vi "Create Detrough Envelope Waveform.vi"(0 "Reference Waveform":T3 {"Runtime Scaling" format="%#_6p"; "Sample Rate" format="%#_6p"; "Burst Length (s)" format="%#_6p"; "PAPR (dB)" format="%.2f"; "Signal Bandwidth (Hz)" format="%#_6p"}, 5 "Detrough Configuration":T1={"Type"=enum."Exponential", "Minimum Voltage (V)"=1.5, "Maximum Voltage (V)"=3.5, "Exponent"=1.2000000476837158}, 11 "error in (no error)":errorcluster) -> (4 "Detrough Envelope Waveform":T3 {"Runtime Scaling" format="%#_6p"; "Sample Rate" format="%#_6p"; "Burst Length (s)" format="%#_6p"; "PAPR (dB)" format="%.2f"; "Signal Bandwidth (Hz)" format="%#_6p"}, 15 "error out":errorcluster)   [LabVIEW 2019, in "Envelope Tracking.lvlib"]
doc: "Creates an envelope waveform utilizing the detrough method."
uses:
  Envelope Tracking.lvlib
  Common/Waveform.ctl
  Typedefs/Detrough Configuration.ctl
  Typedefs/Detrough Type.ctl
  Common/Common.lvlib
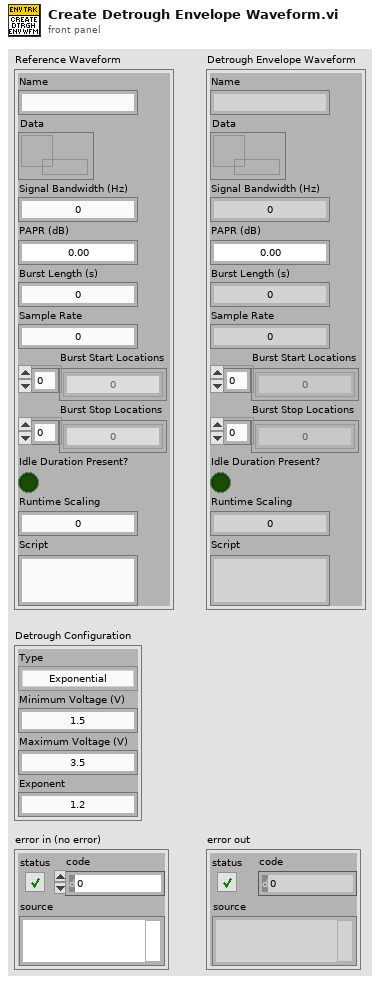
[diagram p1: front panel]
types:
  T1 = typedef "Envelope Tracking.lvlib/Detrough Configuration.ctl" = cluster{"Type":T2, "Minimum Voltage (V)":dbl, "Maximum Voltage (V)":dbl, "Exponent":dbl}
  T2 = typedef "Envelope Tracking.lvlib/Detrough Type.ctl" = enum16{"Exponential", "Cosine", "Power"}
  T3 = typedef "Common.lvlib/Waveform.ctl" = cluster{"Name":string, "Data":refnum<data-value>, "Signal Bandwidth (Hz)":dbl, "PAPR (dB)":dbl, "Burst Length (s)":dbl, "Sample Rate":dbl, "Burst Start Locations":i32[], "Burst Stop Locations":i32[], "Idle Duration Present?":bool, "Runtime Scaling":dbl, "Script":string}
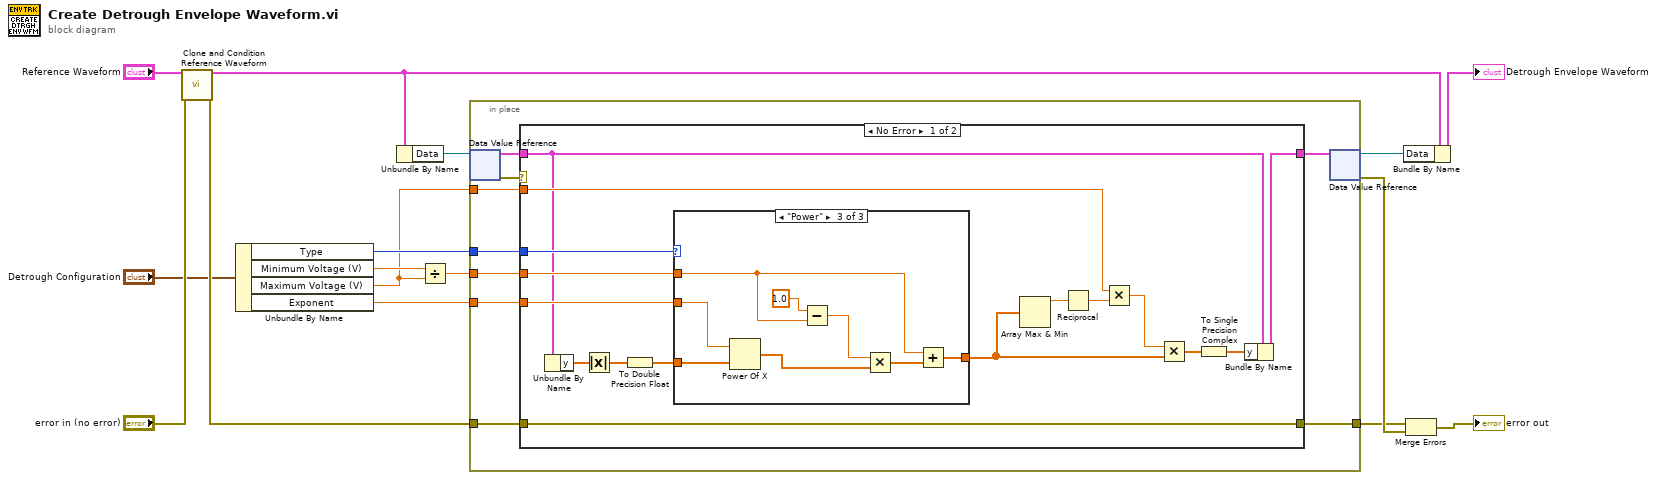
[diagram p0: block diagram]
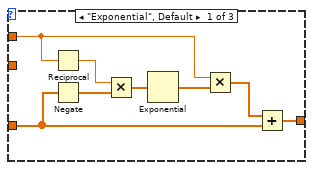
[diagram p2: hidden frame]
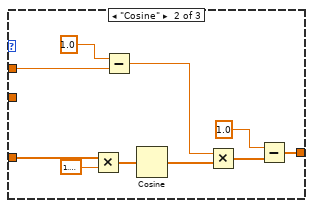
[diagram p3: hidden frame]
diagram:
  n1 = call "Clone and Condition Reference Waveform.vi"("Reference Waveform"="Reference Waveform", "error in (no error)"="error in (no error)") -> ("Conditioned Reference Waveform"=w3:T3, "error out"=w15:errorcluster)  [unwired: 12 in]
  n2 = Unbundle By Name("Detrough Configuration") -> ("Type"=w9:T2, "Minimum Voltage (V)"=w8:dbl, "Maximum Voltage (V)"=w7:dbl, "Exponent"=w6:dbl)
  n3 = Unbundle By Name(w3) -> ("Data"=w2:refnum<data-value>)
  n4 = Divide(x=w8, y=w7) -> (x/y=w10:dbl)
  n5 = in-place {
    in-place-border: w10 -> [w22]
    in-place-border: w9 -> [w21]
    in-place-border: w7 -> [w20]
    in-place-border: w6 -> [w19]
    in-place-border: w15 -> [w24]
    in-place-border: [w23] -> w13
    n6 = in-place-dvr #1(w2) -> (w18:cluster{"t0":dbl, "dt":dbl, "y":csg[]}, w25:errorcluster)
    n7 = case shown="No Error" w25 {
      tunnel: w22 -> [w38 _]
      tunnel: w21 -> [w36 _]
      tunnel: w20 -> [w35 _]
      tunnel: w19 -> [w34 _]
      tunnel: w18 -> [w27 w68]
      tunnel: [w26 w68] -> w17
      tunnel: w24 -> [w41 w69]
      tunnel: [w41 w69] -> w23
      frame No Error {
        n8 = Unbundle By Name(w27) -> ("y"=w33:csg[])
        n9 = Absolute Value(x=w33) -> (abs(x)=w31:sgl[])
        n10 = To Double Precision Float(number=w31) -> (double precision float=w30:dbl[])
        n11 = case shown="\"Power\"" w36 {
          tunnel: w30 -> [w43 w59 w67]
          tunnel: w38 -> [w45 w51 w61]
          tunnel: [w42 w54 w63] -> w32
          tunnel: w34 -> [_ _ w66]
          frame "Exponential", Default {
            n12 = Reciprocal(x=w45) -> (1/x=w47:dbl)
            n13 = Negate(x=w43) -> (-x=w49:dbl[])
            n14 = Multiply(x=w47, y=w49) -> (x*y=w48:dbl[])
            n15 = Exponential(1:w48) -> (0:w46:dbl[])
            n16 = Multiply(x=w45, y=w46) -> (x*y=w44:dbl[])
            n17 = Add(x=w44, y=w43) -> (x+y=w42:dbl[])
          }
          frame "Cosine" {
            n18 = Multiply(x=w59, y=1.5707963267948966) -> (x*y=w58:dbl[])
            n19 = Subtract(x=1.0, y=w51) -> (x-y=w50:dbl)
            n20 = Cosine(x=w58) -> (cos(x)=w57:dbl[])
            n21 = Multiply(x=w50, y=w57) -> (x*y=w55:dbl[])
            n22 = Subtract(x=1.0, y=w55) -> (x-y=w54:dbl[])
          }
          frame "Power" {
            n23 = Power Of X(1:w67, 2:w66) -> (0:w65:dbl[])
            n24 = Subtract(x=1.0, y=w61) -> (x-y=w60:dbl)
            n25 = Multiply(x=w60, y=w65) -> (x*y=w64:dbl[])
            n26 = Add(x=w61, y=w64) -> (x+y=w63:dbl[])
          }
        }
        n27 = Array Max & Min(array=w32) -> (max value=w40:dbl)  [unwired: 3 out]
        n28 = Reciprocal(x=w40) -> (1/x=w39:dbl)
        n29 = Multiply(x=w35, y=w39) -> (x*y=w37:dbl)
        n30 = Multiply(x=w37, y=w32) -> (x*y=w29:dbl[])
        n31 = To Single Precision Complex(1:w29) -> (0:w28:csg[])
        n32 = Bundle By Name(cluster=w27, "y"=w28) -> (w26:cluster{"t0":dbl, "dt":dbl, "y":csg[]})
      }
      frame Error {
      }
    }
    n33 = in-place-dvr #1(w17) -> (w1:refnum<data-value>, w14:errorcluster)
  }
  n34 = Bundle By Name(cluster=w3, "Data"=w1) -> (→"Detrough Envelope Waveform":T3)
  n35 = Merge Errors(w13, w14) -> (→"error out":errorcluster)
